vi "Solenoid - Fill.vi"(8 "Error In":errorcluster, 9 "HEWH MW100 Channel Numbers":T2="011", 10 "Input Valve":T1, 11 "VISA session":refnum<visa-resource-name>="MW100") -> (0 "Error Out":errorcluster, 3 "dup VISA session":refnum<visa-resource-name>)   [LabVIEW 2016]
uses:
  Type Definitions/HEWH MW100 Channel Numbers.ctl
  Type Definitions/HEWH Normally Open Valve Control.ctl
panel:
  out "Message":string
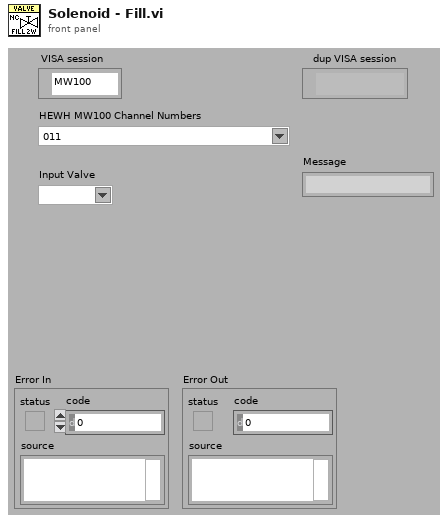
[diagram p1: front panel]
types:
  T1 = typedef "HEWH Normally Open Valve Control.ctl" = string
  T2 = typedef "HEWH MW100 Channel Numbers.ctl" = string
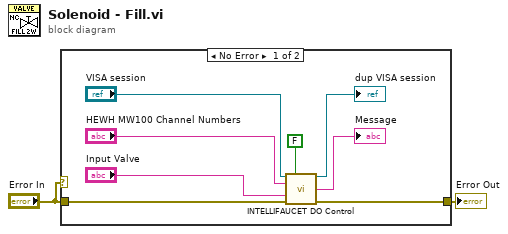
[diagram p0: block diagram]
diagram:
  n1 = case shown="No Error" "Error In" {
    selector: "Error In" -> [_ w11]
    tunnel: "Error In" -> [w8 _]
    tunnel: [w7 w11] -> w2
    frame No Error {
      n2 = call "INTELLIFAUCET DO Control.vi"("VISA session"="VISA session", "Normally Closed Valve?"=FALSE, "HEWH MW100 Channel Numbers"="HEWH MW100 Channel Numbers", "Normally Open Valve"="Input Valve", "Error In"=w8) -> ("dup VISA session"=→"dup VISA session":refnum<visa-resource-name>, "Message"=→"Message":string, "error out"=w7:errorcluster)  [unwired: 7 in, 1 out]
    }
    frame Error {
    }
  }
  "Error Out" <- w2
